vi "Send InitializationData_ZA.vi"(7 "Message Priority (Normal)":T2=enum."Normal", 8 "error in (no error)":errorcluster, 10 "InitializationData":T1, 11 "Message Enqueuer":refnum<class "Message Enqueuer.lvclass">) -> (0 "error out":errorcluster, 3 "Message Enqueuer out":refnum<class "Message Enqueuer.lvclass">)   [LabVIEW 2015, in "InitializationData_ZA Msg.lvclass"]
doc: "This VI sends the message to an actor."
uses:
  InitializationData_ZA Msg.lvclass
  <vilib>/ActorFramework/Message Enqueuer/Message Enqueuer.lvclass
  <vilib>/ActorFramework/Message Enqueuer/Message Priority.ctl
  Zen Analytics/Dependency/Initialize_Cluster.ctl
  Zen Analytics/Zen Analytics.lvclass
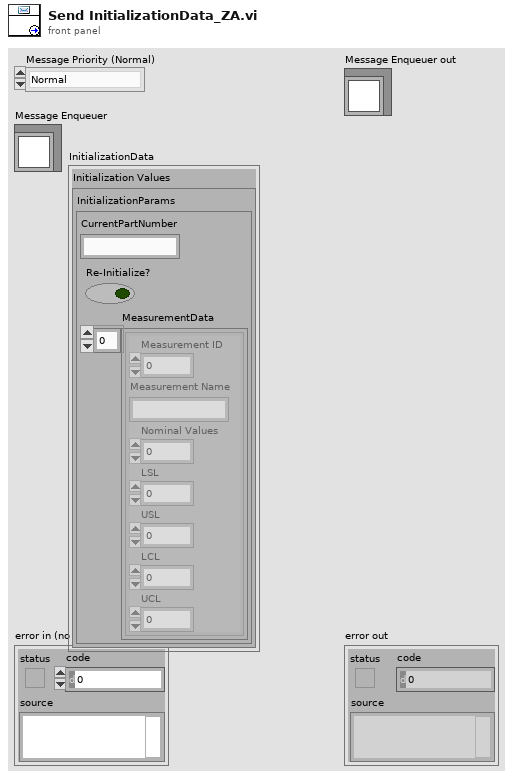
[diagram p1: front panel]
types:
  T1 = typedef "Zen Analytics.lvclass/Initialize_Cluster.ctl" = cluster{"Initialization Values ":cluster{"InitializationParams":cluster{"CurrentPartNumber":string, "Re-Initialize?":bool, "MeasurementData":cluster{"Measurement ID":i32, "Measurement Name":string, "Nominal Values":dbl, "LSL":dbl, "USL":dbl, "LCL":dbl, "UCL":dbl}[]}}}
  T2 = typedef "Actor Framework.lvlib/Message Enqueuer.lvclass/Message Priority.ctl" = enum16{"Low", "Normal", "High"}
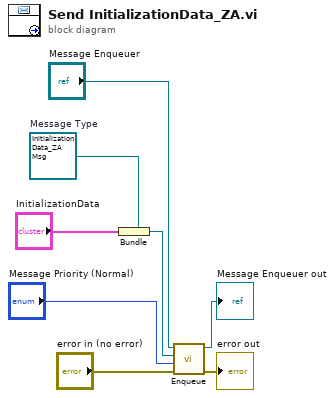
[diagram p0: block diagram]
diagram:
  w5 = refnum<class "InitializationData_ZA Msg.lvclass"> refnum  # Message Type
  n1 = Bundle(cluster=w5, "InitializationData") -> (w4:refnum<class "InitializationData_ZA Msg.lvclass">)
  n2 = call <vilib>:"Enqueue.vi"("error in (no error)"="error in (no error)", "Message Priority (Normal)"="Message Priority (Normal)", "Message"=w4, "Message Enqueuer in"="Message Enqueuer") -> ("error out"=→"error out":errorcluster, "Message Enqueuer out"=→"Message Enqueuer out":refnum<class "Message Enqueuer.lvclass">)  [unwired: 6 in]
